vi "acquiring data.vi"() -> ()   [LabVIEW 2014]
uses:
  <vilib>/rvi/Emulation/niFpgaGetClockAttributes.vi
  <vilib>/rvi/Emulation/niFpgaSctlEmulationGetInTimedLoop.vi
  <vilib>/rvi/Emulation/niFpgaEmulationReportErrorSimple.vi
  <vilib>/rvi/eio/common/nirviEmuTemplateMethod_errors.vi
  <vilib>/rvi/interface/RandomDataEmulation/niFpgaRandomDataHandleErrors.vi
  <vilib>/rvi/Emulation/niFpgaCriticalErrorInLSC.vi
  <vilib>/eio/EIONode/EIONode.xnode
  <vilib>/rvi/DataTransferAndStorage/Container/XNode/niFpgaContainer.xnode
  <vilib>/rvi/interface/RandomDataEmulation/nirviRandomDataFpgaReadWriteTemplate.vi
panel:
  in  "Loop Period (ticks)":u32 caption="Count(Ticks)"
  in  "Stop Button":bool
  out "FIFO Full?":bool
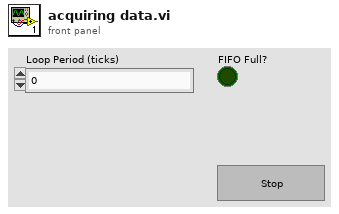
[diagram p1: front panel]
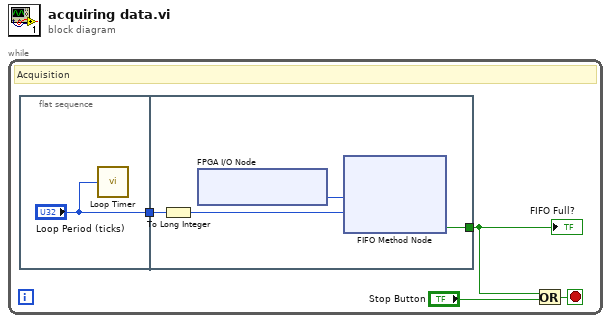
[diagram p0: block diagram]
diagram:
  n1 = while {
    stop <- w3 stop-if-true
    # "Acquisition"
    n2 = flat-sequence {
      tunnel: ["Loop Period (ticks)"] -> w4
      tunnel: w4 -> [w8]
      tunnel: [w7] -> w1
      frame #0 {
        n3 = call "Loop Timer"("Count(Ticks)"="Loop Period (ticks)") -> ()  [unwired: 1 out]
      }
      frame #1 {
        n4 = To Long Integer(number=w8) -> (32bit integer=w9:i32)
        n5 = xnode "FPGA I/O Node"() -> ("ConnectorC/AI0"=w6:i16)  [unwired: 1 in, 1 out]
        n6 = xnode ("FIFO Method Node")("Element"=w6, "Timeout"=w9) -> ("Timed Out?"=w7:bool)  [unwired: 1 in, 1 out]
      }
    }
    n7 = Or(x=w1, y="Stop Button") -> (x .or. y?=w3:bool)
    "FIFO Full?" <- w1
  }
